vi "ErrCode.vi"(11 "error IO":errorcluster) -> (3 "布尔":bool)   [LabVIEW 2011]
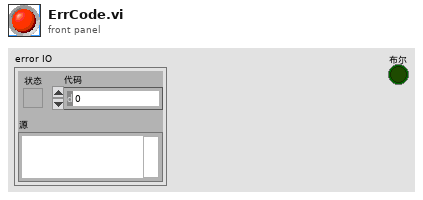
[diagram p1: front panel]
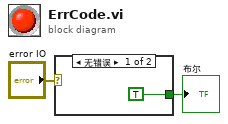
[diagram p0: block diagram]
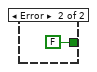
[diagram p2: hidden frame]
diagram:
  n1 = case shown="无错误" "error IO" {
    tunnel: [TRUE FALSE] -> w1
    frame No Error {
    }
    frame Error {
    }
  }
  "布尔" <- w1
